vi "Set Multiple Tags.vi"(8 "error in (no error)":errorcluster, 10 "Cluster":variant, 11 "uData in":refnum<class "uData.lvclass">) -> (0 "error out":errorcluster, 3 "uData out":refnum<class "uData.lvclass">, 4 "replaced?":bool, 6 "replaced tags":string[](array[string]))   [LabVIEW 2023, in "uLib.lvlib" / "uData.lvclass"]
doc: "Wire in a cluster. The cluster will be broken into individual elements, each element is used to append a new tag or replace an existing tag. \nNested clusters use a label[dot]sublabel notation. \n\nThis method returns an error if a naming conflict exists (e.g: a cluster with a 'nums.one' element and another cluster element labelled 'nums' that nests a 'one' element)\n\nDo NOT use for handling data at high rates. This VI does not support inlining. The basic accessor method are more efficient for recurring high rate VI calls."
uses:
  uData.lvclass
  uData.lvclass/uData.ctl
  Inline Write.vi
  Condition Tag Names.vi
  Condition Tag Name.vi
  Blank Key Reserved String.vi
  <vilib>/Utility/error.llb/Error Cluster From Error Code.vi
  <vilib>/ErrorRing/Error Ring.xnode
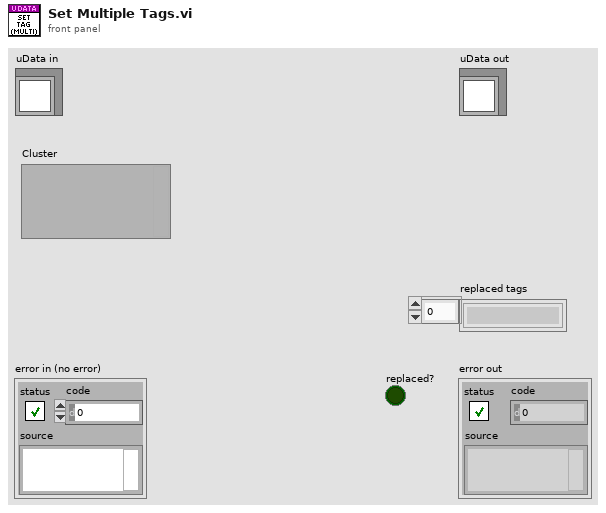
[diagram p1: front panel]
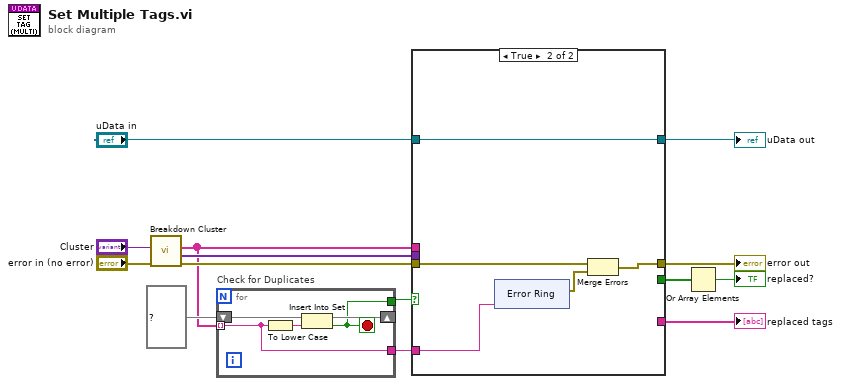
[diagram p0: block diagram]
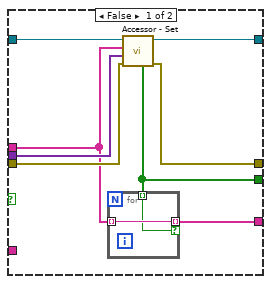
[diagram p2: hidden frame]
diagram:
  n1 = call "Breakdown Cluster.vi"("error in (no error)"="error in (no error)", "Cluster"="Cluster") -> ("error out"=w9:errorcluster, "values"=w8:variant[], "tags"=w3:string[])  [unwired: 7 in]
  n2 = for "Check for Duplicates" {
    shift-right: [w18] -> _
    shift-left: set{string} {} ("set") -> [w19]
    tunnel: w3 -> [w15] mode=indexing
    tunnel: [w16] -> w2
    tunnel: [w15] -> w1
    stop <- w16 stop-if-true
    n3 = To Lower Case(string=w15) -> (all lower case string=w17:string)
    n4 = Insert Into Set(10:w17, 11:w19) -> (2:w16:bool, 3:w18:set{string})
  }
  n5 = case shown="True" w2 {
    tunnel: [w27 w32] -> w14
    tunnel: [w26 w34] -> w13
    tunnel: "uData in" -> [w25 w34]
    tunnel: w9 -> [w24 w33]
    tunnel: w8 -> [w23 _]
    tunnel: [w20 _] -> w7
    tunnel: [w21 _] -> w5
    tunnel: w3 -> [w22 _]
    tunnel: w1 -> [_ w30]
    frame False {
      n6 = call "Accessor - Set.vi"("error in (no error)"=w24, "values"=w23, "keys"=w22, "uData in"=w25) -> ("error out"=w27:errorcluster, "uData out"=w26:refnum<class "uData.lvclass">, "replaced?"=w20:bool[])  [unwired: 5 in]
      n7 = for {
        tunnel: w22 -> [w29] mode=indexing
        tunnel: [w29] -> w21 mode=indexing if=w28
        tunnel: w20 -> [w28] mode=indexing
      }
    }
    frame True {
      n8 = xnode ("Error Ring")("parameter 0"=w30) -> ("error out"=w31:errorcluster)
      n9 = Merge Errors(w33, w31) -> (w32:errorcluster)
    }
  }
  "error out" <- w14
  "uData out" <- w13
  "replaced tags" <- w5
  n10 = Or Array Elements(Boolean array=w7) -> (logical OR=→"replaced?":bool)
